vi "ReadSectionPathKeys.vi"(8 "error in (no error)":errorcluster, 9 "section":string, 10 "Workspace Path":path, 11 "Refnum in":T1) -> (0 "error out":errorcluster, 2 "Paths":path[](array[path]), 3 "refnum out":T1)   [LabVIEW 2019, in "DepsWatch.lvlib"]
uses:
  DepsWatch.lvlib
  <vilib>/Utility/config.llb/Config Data RefNum.ctl
  <vilib>/Utility/config.llb/NI_LVConfig.lvlib
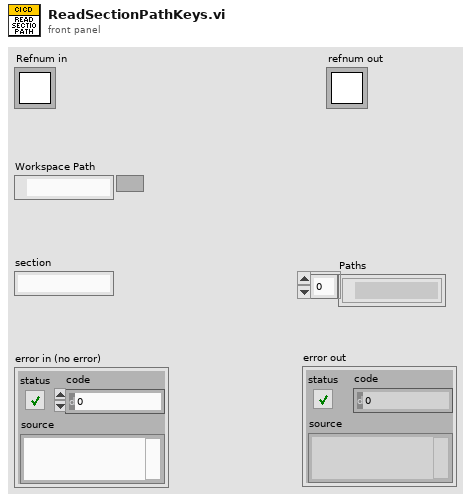
[diagram p1: front panel]
types:
  T1 = typedef "NI_LVConfig.lvlib/Config Data RefNum.ctl" = refnum<k1>
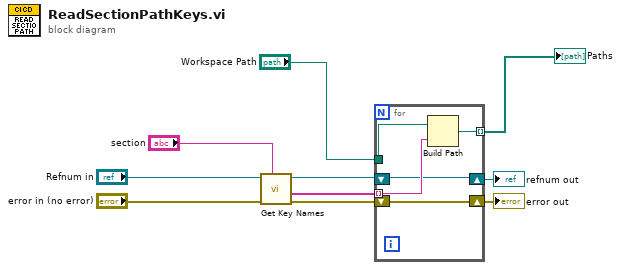
[diagram p0: block diagram]
diagram:
  n1 = call <vilib>:"Get Key Names.vi"("section"="section", "error in (no error)"="error in (no error)", "refnum"="Refnum in") -> ("error out"=w7:errorcluster, "key names"=w8:string[], "refnum out"=w6:T1)  [unwired: 5 in, 1 out]
  n2 = for {
    shift-right: [w13] -> w1
    shift-left: w7 -> [w13]
    tunnel: w8 -> [w14] mode=indexing
    tunnel: "Workspace Path" -> [w15]
    tunnel: [w12] -> w10 mode=indexing
    shift-right: [w11] -> w2
    shift-left: w6 -> [w11]
    n3 = Build Path(base path=w15, name or relative path=w14) -> (appended path=w12:path)
  }
  "Paths" <- w10
  "refnum out" <- w2
  "error out" <- w1
